vi "ImpulseAnalyzer.vi"() -> ()   [LabVIEW 2015]
uses:
  <vilib>/express/express analysis/Spectral/Block/exnSpectralBlock spectral measurements RMS poly.vi
  <vilib>/express/express analysis/Spectral/Block/exnSpectralBlock spectral measurements RMS WFM.vi
  <vilib>/express/express analysis/Spectral/XNode/ExpressSpectralMeasurementsBlockNode.xnode
panel:
  in  "stop":bool
  in  "error in":errorcluster
  out "error out":errorcluster
  out "FFT":cluster{"f0":dbl, "df":dbl, "magnitude":dbl[]}(graph)
  out "Average Signal":waveform(dbl)(graph)
  in  "Time (ms)":dbl
  in  "Averages":i32
  in  "rate":dbl=1000.0
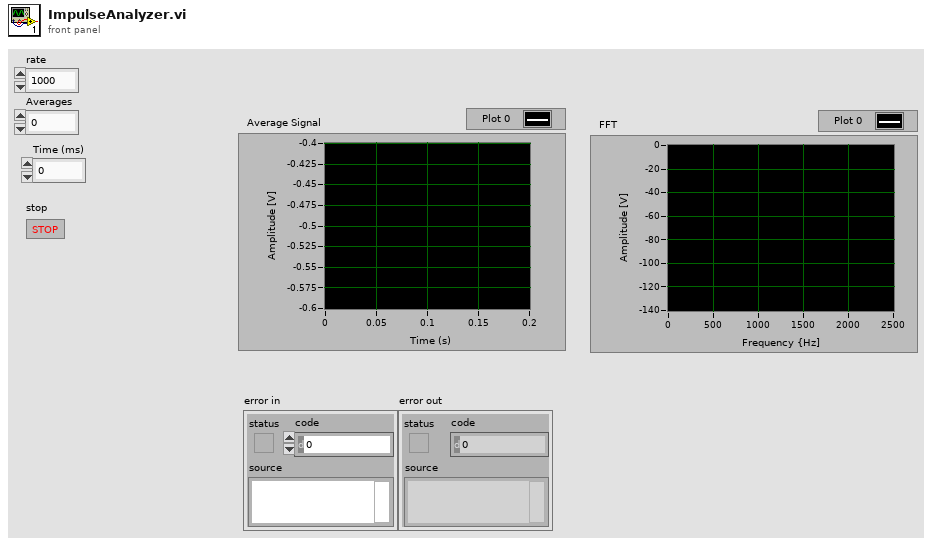
[diagram p1: front panel]
types:
  T1 = cluster{"averaging mode":u16, "weighting mode":u16, "number of averages":u32}
  T2 = cluster{"dB On (F)":bool, "unwrap phase (F)":bool, "convert to degree (F)":bool}
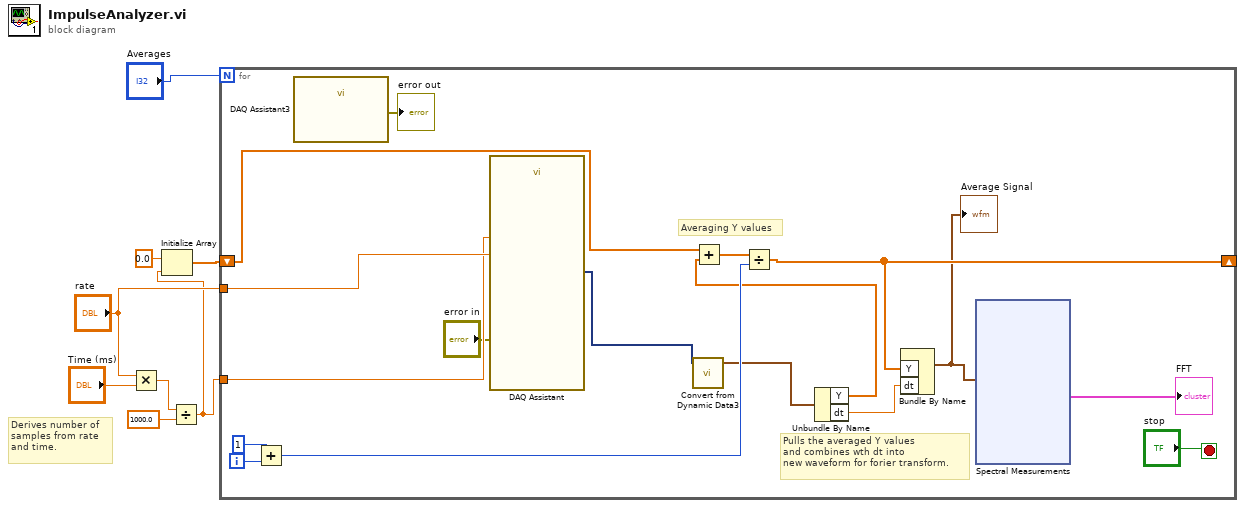
[diagram p0: block diagram]
diagram:
  # "Derives number of \nsamples from rate \nand time."
  n1 = Multiply(x="rate", y="Time (ms)") -> (x*y=w4:dbl)
  n2 = Divide(x=w4, y=1000.0) -> (x/y=w2:dbl)
  n3 = Initialize Array(0.0 ("element"), w2) -> (w8:dbl[])
  n4 = for {
    N: "Averages" -> [_]
    shift-right: [w14] -> _
    shift-left: w8 -> [w25]
    tunnel: "rate" -> [w24]
    tunnel: w2 -> [w23]
    i -> [w21]
    stop <- "stop" stop-if-true
    # "Averaging Y values"
    # "Pulls the averaged Y values\nand combines wth dt into \nnew waveform for forier transform."
    n5 = Add(x=1, y=w21) -> (x+y=w19:i32)
    n6 = call "DAQ Assistant3"() -> ("error out"=→"error out":errorcluster)  [unwired: 18 in, 1 out]
    n7 = call "DAQ Assistant"("rate"=w24, "number of samples"=w23, "error in"="error in") -> ("data"=w18:dynamicdata)  [unwired: 14 in, 2 out]
    n8 = call "Convert from Dynamic Data3"("Dynamic Data Type"=w18) -> ("Waveform"=w17:waveform(dbl))  [unwired: 3 in]
    n9 = Unbundle By Name(w17) -> ("Y"=w15:dbl[], "dt"=w16:dbl)
    n10 = Add(x=w25, y=w15) -> (x+y=w22:dbl[])
    n11 = Divide(x=w22, y=w19) -> (x/y=w14:dbl[])
    n12 = Bundle By Name("Y"=w14, "dt"=w16) -> (w13:waveform(dbl))  [unwired: 1 in]
    "Average Signal" <- w13
    n13 = xnode "Spectral Measurements"("Signals"=w13) -> ("FFT - (RMS)"=→"FFT":cluster{"f0":dbl, "df":dbl, "magnitude":dbl[]})  [unwired: 1 in, 2 out]
  }
